vi "AFG1022Waveforms.VI"() -> ()   [LabVIEW 2017]
uses:
  <vilib>/measure/NI_MABase.lvlib
panel:
  in  "amplitude":dbl=1.0 caption="幅值" format="%0.2p"
  in  "VISA资源名称":refnum<visa-resource-name>
  in  "频率":dbl
  in  "signal type":T1(ring) caption="信号类型"
  out "波形图":waveform(dbl)(graph)
  # "输出波形信息"
  # "Hz"
  # "V"
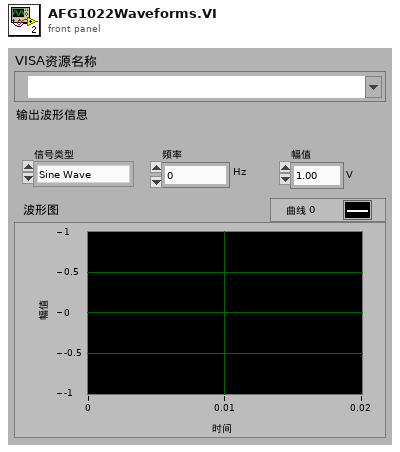
[diagram p1: front panel]
types:
  T1 = enum16{"Sine Wave", "Triangle Wave", "Square Wave", "Sawtooth Wave"}
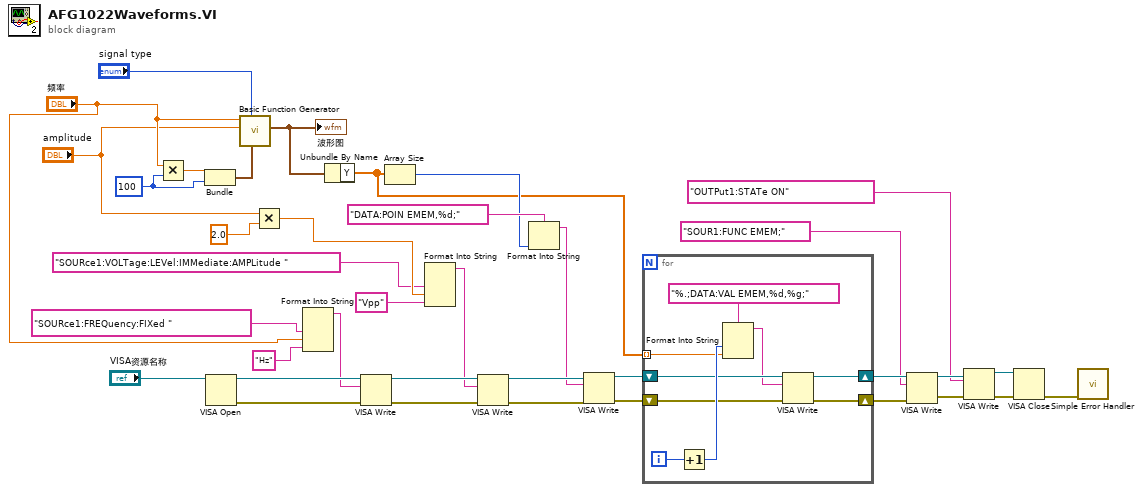
[diagram p0: block diagram]
diagram:
  w3 = 100
  n1 = Multiply(x="频率", y=w3) -> (x*y=w16:dbl)
  n2 = Bundle(w16, w3) -> (w15:cluster{dbl, i32})  [unwired: 1 in]
  n3 = VISA Open(VISA resource name="VISA资源名称") -> (VISA resource name=w32:refnum<visa-resource-name>, error out=w31:errorcluster)  [unwired: 4 in]
  n4 = call <vilib>:"Basic Function Generator.vi"("sampling info"=w15, "signal type"="signal type", "amplitude"="amplitude", "frequency"="频率") -> ("signal out"=w2:waveform(dbl))  [unwired: 5 in, 2 out]
  "波形图" <- w2
  n5 = Multiply(x="amplitude", y=2.0) -> (x*y=w5:dbl)
  n6 = Format Into String("SOURce1:FREQuency:FIXed " ("写入缓冲区"), "频率", "Hz" ("输入 3")) -> (resulting string=w8:string)  [unwired: 3 in, 1 out]
  n7 = Unbundle By Name(w2) -> ("Y"=w26:dbl[])
  n8 = VISA Write(VISA resource name=w32, write buffer=w8, error in (no error)=w31) -> (VISA resource name out=w37:refnum<visa-resource-name>, error out=w36:errorcluster)  [unwired: 1 out]
  n9 = Array Size(array=w26) -> (size(s)=w29:i32)
  n10 = Format Into String("SOURce1:VOLTage:LEVel:IMMediate:AMPLitude " ("写入缓冲区"), w5, "Vpp" ("输入 3")) -> (resulting string=w12:string)  [unwired: 3 in, 1 out]
  n11 = VISA Write(VISA resource name=w37, write buffer=w12, error in (no error)=w36) -> (VISA resource name out=w28:refnum<visa-resource-name>, error out=w27:errorcluster)  [unwired: 1 out]
  n12 = Format Into String(format string="DATA:POIN EMEM,%d;", w29) -> (resulting string=w14:string)  [unwired: 2 in, 1 out]
  n13 = VISA Write(VISA resource name=w28, write buffer=w14, error in (no error)=w27) -> (VISA resource name out=w1:refnum<visa-resource-name>, error out=w25:errorcluster)  [unwired: 1 out]
  n14 = for {
    tunnel: w26 -> [w43] mode=indexing
    shift-right: [w40] -> w24
    shift-left: w1 -> [w42]
    shift-right: [w39] -> w23
    shift-left: w25 -> [w41]
    i -> [w45]
    n15 = Increment(x=w45) -> (x+1=w44:i32)
    n16 = Format Into String(format string="%.;DATA:VAL EMEM,%d,%g;", w44, w43) -> (resulting string=w38:string)  [unwired: 2 in, 1 out]
    n17 = VISA Write(VISA resource name=w42, write buffer=w38, error in (no error)=w41) -> (VISA resource name out=w40:refnum<visa-resource-name>, error out=w39:errorcluster)  [unwired: 1 out]
  }
  n18 = VISA Write(VISA resource name=w24, write buffer="SOUR1:FUNC EMEM;" ("写入缓冲区"), error in (no error)=w23) -> (VISA resource name out=w21:refnum<visa-resource-name>, error out=w20:errorcluster)  [unwired: 1 out]
  n19 = VISA Write(VISA resource name=w21, write buffer="OUTPut1:STATe ON" ("写入缓冲区"), error in (no error)=w20) -> (VISA resource name out=w18:refnum<visa-resource-name>, error out=w17:errorcluster)  [unwired: 1 out]
  n20 = VISA Close(VISA resource name=w18, error in (no error)=w17) -> (error out=w35:errorcluster)
  n21 = call <vilib>:"Simple Error Handler.vi"("error in (no error)"=w35) -> ()  [unwired: 4 in, 5 out]
